vi "Insert While Loop.vi"(8 "error in (no error)":errorcluster, 10 "Insert While Loop":T1, 11 "Test Executive Builder Model in":refnum<class "Test Executive Builder Model.lvclass">) -> (0 "error out":errorcluster, 3 "Test Executive Builder Model out":refnum<class "Test Executive Builder Model.lvclass">, 5 "Unique ID out":string)   [LabVIEW 2019, in "Test Executive Builder Model.lvclass"]
uses:
  <vilib>/gpm_packages/@cs/Test-executive-builder/Source/Test Executive Builder Model/Test Executive Builder Model/Test Executive Builder Model.lvclass
  C:/Program Files/National Instruments/LabVIEW 2019/vi.lib/ActorFramework/Actor/Actor.lvclass
  <vilib>/gpm_packages/@cs/Test-executive-builder/Source/Application Dependencies/Insert While Loop.ctl
  <vilib>/gpm_packages/@cs/Test-executive-builder/Source/Test Executive Builder Model/Test Executive Builder Model/Test Executive Builder Model.lvclass/Test Executive Builder Model.ctl
  <vilib>/ActorFramework/Actor/Actor.lvclass/Actor.ctl
  <vilib>/ActorFramework/Message Enqueuer/Message Enqueuer.lvclass/Message Enqueuer.ctl
  <vilib>/ActorFramework/Message Enqueuer/Init from Existing Queue.vi
  <vilib>/ActorFramework/Message Enqueuer/Enqueue.vi
  <vilib>/gpm_packages/@cs/Test-executive-builder/Source/Test Executive Builder Model/Test Executive Builder Model Messages/Redraw Tree Msg/Redraw Tree Msg.lvclass
  C:/Program Files/National Instruments/LabVIEW 2019/vi.lib/ActorFramework/Message/Message.lvclass
  <vilib>/ActorFramework/Message Priority Queue/Priority Enqueue.vi
  <vilib>/ActorFramework/Message Enqueuer/Message Enqueuer.lvclass
  <vilib>/gpm_packages/@cs/test-executive/Source/Test Executive/TestExecutive Ref/TestExecutive Ref.lvclass
  <vilib>/ActorFramework/Actor/Actor.lvclass
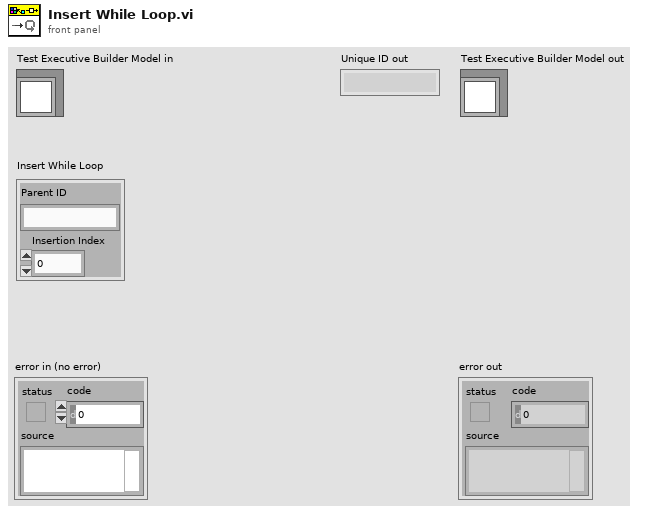
[diagram p1: front panel]
types:
  T1 = typedef "Insert While Loop.ctl" = cluster{"Parent ID":string, "Insertion Index":i32}
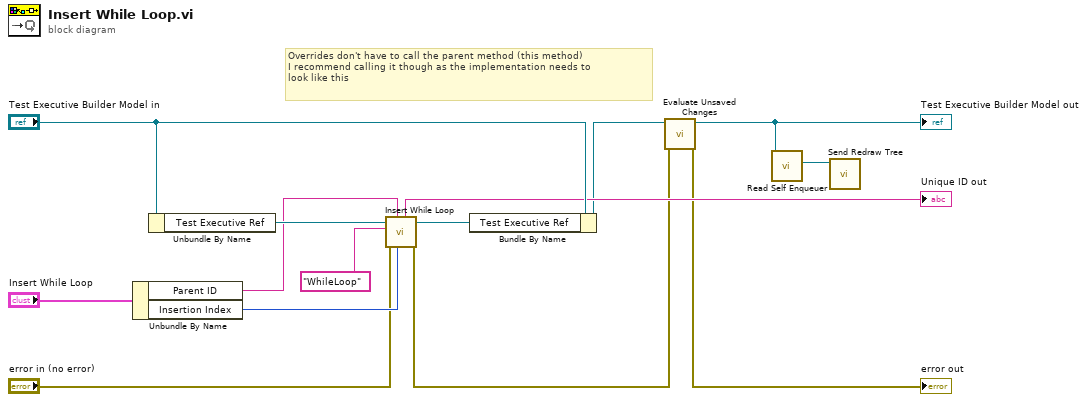
[diagram p0: block diagram]
diagram:
  # "Overrides don't have to call the parent method (this method)\nI recommend calling it though as the implementation needs to\nlook like this"
  n1 = Unbundle By Name("Insert While Loop") -> ("Parent ID"=w11:string, "Insertion Index"=w12:i32)
  n2 = Unbundle By Name("Test Executive Builder Model in") -> ("Test Executive Ref"=w14:refnum<data-value>)
  n3 = call <vilib>:"Insert While Loop.vi"("Insertion Index"=w12, "Parent ID"=w11, "error in (no error)"="error in (no error)", "Name"="WhileLoop" ("format string"), "Test Executive Ref"=w14) -> ("error out"=w2:errorcluster, "Test Executive Ref out"=w9:refnum<data-value>, "Unique ID out"=→"Unique ID out":string)  [unwired: 3 in, 1 out]
  n4 = Bundle By Name(cluster="Test Executive Builder Model in", "Test Executive Ref"=w9) -> (w4:refnum<class "Test Executive Builder Model.lvclass">)
  n5 = call-dynamic "Evaluate Unsaved Changes.vi"("error in (no error)"=w2, "Test Executive Builder Model in"=w4) -> ("error out"=→"error out":errorcluster, "Test Executive Builder Model out"=w3:refnum<class "Test Executive Builder Model.lvclass">)  [unwired: 8 in]
  "Test Executive Builder Model out" <- w3
  n6 = call <vilib>:"Read Self Enqueuer.vi"("Actor"=w3) -> ("Self Enqueuer"=w6:refnum<class "Message Enqueuer.lvclass">)  [unwired: 10 in]
  n7 = call <vilib>:"Send Redraw Tree.vi"("Message Enqueuer"=w6) -> ()  [unwired: 9 in, 2 out]
